vi "Test Method Result Published.vi"(8 "error in (no error)":errorcluster, 11 "Result Observation Test In":refnum<class "Result Observation Test.lvclass">) -> (0 "error out":errorcluster, 3 "Result Observation Test Out":refnum<class "Result Observation Test.lvclass">)   [LabVIEW 2020, in "Result Observation Test.lvclass"]
uses:
  Result Observation Test.lvclass
  Result Observation Test.lvclass/Result Observation Test.ctl
  Mock Result Observer/Mock Result Observer.lvclass
  source/LUnit Test Case.lvclass
  Test Doubles/Test Case Test Double/Test Case Test Double.lvclass
  Test Doubles/Test Case Test Double/Methods.ctl
  source/Core/Result/Type.ctl
  source/Core/Result/Result.lvlib
  <vilib>/Astemes/LUnit/Test Case.lvclass
  source/Framework/Single Thread Test Runner/Single Thread Test Runner.lvclass
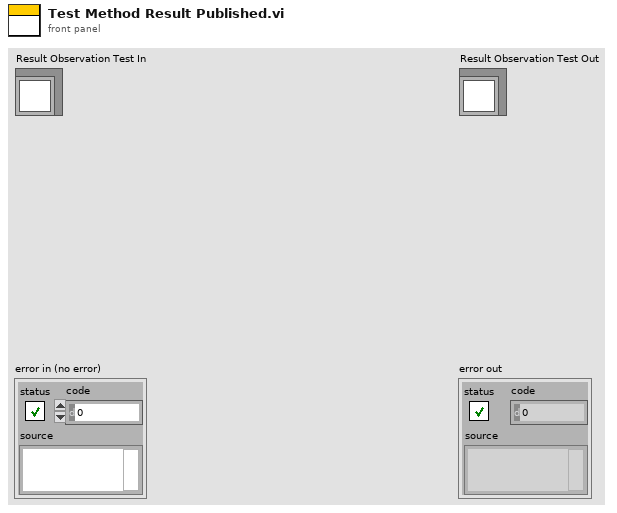
[diagram p1: front panel]
types:
  T1 = typedef "Result.lvlib/Type.ctl" = enum16{"Test Case", "Test Suite", "Test Run", "Pass", "Fail", "Skip", "Pass if", "Fail if", "Pass if Error", "Fail if Error", "Pass if Equal", "Fail if Equal"}
  T2 = typedef "Test Case Test Double.lvclass/Methods.ctl" = enum16{"Test Failing Test.vi", "Test Passing Test.vi", "Test Error Test.vi", "Test Skip Test.vi", "Test Passing Pass If Test.vi", "Test Failing Pass If Test.vi", "Test Failing Fail If Test.vi", "Test Passing Fail If Test.vi", "Test Passing Pass If Error Test.vi", "Test Failing Pass If Error Test.vi", "Test Passing Fail If Error Test.vi", "Test Failing Fail If Error Test.vi", "Test Passing Pass If Equal Test.vi", "Test Failing Pass If Equal Test.vi", "Test Failing Fail If Equal Test.vi", "Test Passing Fail If Equal Test.vi", "Freezing Test.vi", "Test Pass on Expected Error Code.vi", "Test Error on Unexpected Error Code.vi", "Test Fail on Expected Error Code.vi", "Test Error when Fail on Unexpected Error Code.vi", "Test Pass on Expected Element in Array.vi", "Test Fail on Expected Element Not in Array.vi", "Test Pass on Expected Element in Set.vi", "Test Fail on Expected Element Not in Set.vi", "Test Pass on Expected Element in Map.vi", "Test Fail on Expected Element Not in Map.vi", "Test Fail on Unexpected Element in Array.vi", "Test Pass on Unexpected Element Not in Array.vi", "Test Fail if Unexpected Element in Set.vi", "Test Pass if Unexpected Element Not in Set.vi", "Test Fail if Unexpected Element in Map.vi", "Test Pass if Unexpected Element Not in Map.vi", "Test Pass on Expected Element in Array of Clusters.vi", "Test Pass on Expected Element Not in Array of Clusters.vi", "Test Matching String Test.vi", "Test Not Matching String Test.vi", "Verify Passing.vi", "Without Prefix.vi", "Private VI.vi"}
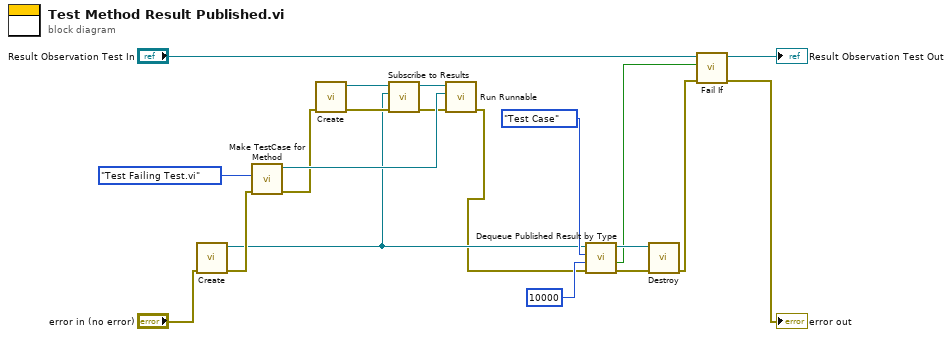
[diagram p0: block diagram]
diagram:
  n1 = call "Create.vi"("error in (no error)"="error in (no error)") -> ("error out"=w14:errorcluster, "Mock Result Observer out"=w3:refnum<class "Mock Result Observer.lvclass">)  [unwired: 9 in]
  n2 = call "Make TestCase for Method.vi"("error in (no error)"=w14, "Test Method"=Methods."Test Failing Test.vi") -> ("error out"=w1:errorcluster, "LUnit Test Case V2 out"=w8:refnum<class "LUnit Test Case.lvclass">)  [unwired: 8 in]
  n3 = call "Create.vi"("error in (no error)"=w1) -> ("error out"=w6:errorcluster, "Single Thread Test Runner out"=w7:refnum<class "Single Thread Test Runner.lvclass">)  [unwired: 9 in]
  n4 = call-dynamic "Subscribe to Results.vi"("error in (no error)"=w6, "Result Observer"=w3, "Single Thread Test Runner In"=w7) -> ("error out"=w4:errorcluster, "Single Thread Test Runner Out"=w5:refnum<class "Single Thread Test Runner.lvclass">)  [unwired: 7 in]
  n5 = call-dynamic "Run Runnable.vi"("error in (no error)"=w4, "Runnable"=w8, "Single Thread Test Runner In"=w5) -> ("error out"=w2:errorcluster)  [unwired: 7 in, 1 out]
  n6 = call "Dequeue Published Result by Type.vi"("error in (no error)"=w2, "timeout in ms"=10000 ("timeout in ms (-1)"), "Result Type"=Type."Test Case", "Mock Result Observer In"=w3) -> ("error out"=w18:errorcluster, "timed out?"=w11:bool, "Mock Result Observer Out"=w19:refnum<class "Mock Result Observer.lvclass">)  [unwired: 4 in, 1 out]
  n7 = call "Destroy.vi"("error in (no error)"=w18, "Mock Result Observer in"=w19) -> ("error out"=w10:errorcluster)  [unwired: 8 in, 1 out]
  n8 = call <vilib>:"Fail If.vi"("error in (no error)"=w10, "Fail?"=w11, "LUnit Test Case In"="Result Observation Test In") -> ("error out"=→"error out":errorcluster, "LUnit Test Case Out"=→"Result Observation Test Out":refnum<class "Result Observation Test.lvclass">)  [unwired: 7 in]
